vi "recalculate_n_tacking_points.vi"(1 "In tacking?":bool, 2 "Calculate tacking points?":bool) -> (0 "Calculate n?":bool)   [LabVIEW 2013]
doc: "We should recalculate the number of tacks if we have just started an upwind sequence or if we're changing in or out of a tack"
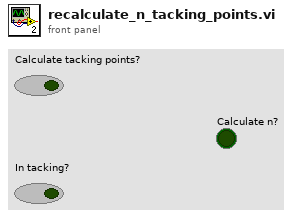
[diagram p1: front panel]
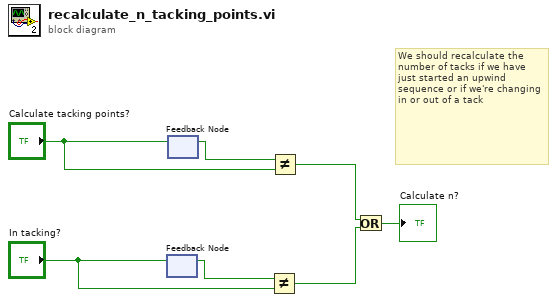
[diagram p0: block diagram]
diagram:
  # "We should recalculate the number of tacks if we have just started an upwind sequence or if we're changing in or out of a tack"
  n1 = feedback #1() -> (w5:bool)  [unwired: 1 in]
  n2 = feedback-in #1("In tacking?") -> ()
  n3 = feedback-in #2("Calculate tacking points?") -> ()
  n4 = feedback #2() -> (w7:bool)  [unwired: 1 in]
  n5 = Not Equal?(x=w5, y="In tacking?") -> (x != y?=w2:bool)
  n6 = Not Equal?(x=w7, y="Calculate tacking points?") -> (x != y?=w3:bool)
  n7 = Or(x=w3, y=w2) -> (x .or. y?=→"Calculate n?":bool)
